vi "Move.vi"(10 "P1":bool, 11 "Circular Buffer in":refnum<class "Circular Buffer.lvclass">) -> (3 "Circular Buffer out":refnum<class "Circular Buffer.lvclass">)   [LabVIEW 2021, in "d20.lvlib" / "Circular Buffer.lvclass"]
uses:
  Circular Buffer.lvclass
  Circular Buffer.lvclass/Circular Buffer.ctl
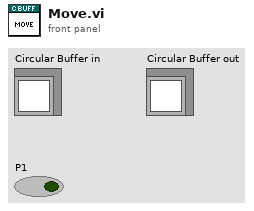
[diagram p1: front panel]
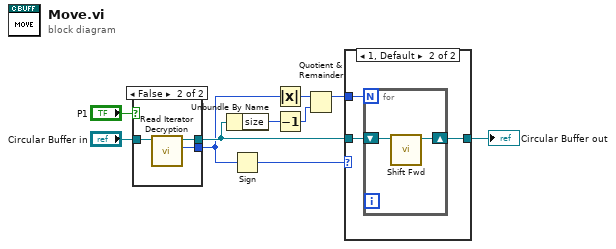
[diagram p0: block diagram]
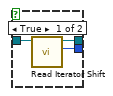
[diagram p2: hidden frame]
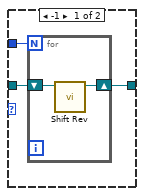
[diagram p3: hidden frame]
diagram:
  n1 = case shown="False" "P1" {
    tunnel: "Circular Buffer in" -> [w13 w16]
    tunnel: [w12 w15] -> w7
    tunnel: [w11 w14] -> w5
    frame True {
      n2 = call "Read Iterator Shift.vi"("Circular Buffer in"=w13) -> ("shift"=w11:i64, "Circular Buffer out"=w12:refnum<class "Circular Buffer.lvclass">)  [unwired: 9 in]
    }
    frame False {
      n3 = call "Read Iterator Decryption.vi"("Circular Buffer in"=w16) -> ("Decryption"=w14:i64, "Circular Buffer out"=w15:refnum<class "Circular Buffer.lvclass">)  [unwired: 9 in]
    }
  }
  n4 = Unbundle By Name(w7) -> ("size"=w6:i64)
  n5 = Sign(1:w5) -> (0:w8:i64)
  n6 = Absolute Value(x=w5) -> (abs(x)=w4:i64)
  n7 = Decrement(x=w6) -> (x-1=w3:i64)
  n8 = Quotient & Remainder(x=w4, y=w3) -> (x-y*floor(x/y)=w2:i64)  [unwired: 1 out]
  n9 = case shown="1, Default" w8 {
    tunnel: [w19 w24] -> w9
    tunnel: w7 -> [w18 w23]
    tunnel: w2 -> [w17 w22]
    frame -1 {
      n10 = for {
        N: w17 -> [_]
        shift-right: [w20] -> w19
        shift-left: w18 -> [w21]
        n11 = call "Shift Rev.vi"("Circular Buffer in"=w21) -> ("Circular Buffer out"=w20:refnum<class "Circular Buffer.lvclass">)  [unwired: 10 in]
      }
    }
    frame 1, Default {
      n12 = for {
        N: w22 -> [_]
        shift-right: [w25] -> w24
        shift-left: w23 -> [w26]
        n13 = call "Shift Fwd.vi"("Circular Buffer in"=w26) -> ("Circular Buffer out"=w25:refnum<class "Circular Buffer.lvclass">)  [unwired: 10 in]
      }
    }
  }
  "Circular Buffer out" <- w9
